vi "Driver VI Template Name.vi"(11 "CD Template":refnum<class "NIVS_Inline HW Interface.lvclass">) -> (2 "Driver VI Template Name":string)   [LabVIEW 2016, in "NIVS_Inline HW Interface.lvclass"]
uses:
  NIVS_Inline HW Interface.lvclass
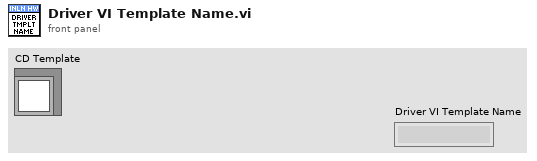
[diagram p1: front panel]
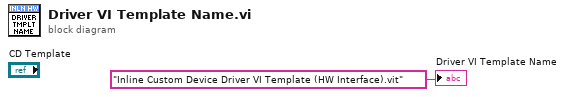
[diagram p0: block diagram]
diagram:
  "Driver VI Template Name" <- "Inline Custom Device Driver VI Template (HW Interface).vit" ("Driver VI Template Name")
